vi "Get Comment.vi"(8 "error in (no error)":errorcluster, 11 "Device in":refnum<class "Device.lvclass">) -> (0 "error out":errorcluster, 2 "Comment":string, 3 "Device out":refnum<class "Device.lvclass">)   [LabVIEW 2020, in "HAL.lvlib" / "Device.lvclass"]
uses:
  Device.lvclass
  Device.lvclass/Device.ctl
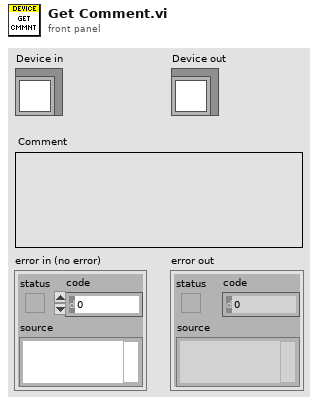
[diagram p1: front panel]
types:
  T1 = typedef "HAL.lvlib/Device.lvclass/Ref Data.ctl" = cluster{"Config Keys":string[], "Config Values":string[], "Cal Expires":timestamp, "Name":string, "Comment":string, "State":T2, "Error":errorcluster}
  T2 = typedef "HAL.lvlib/Device.lvclass/Device State.ctl" = enum16{"Uninitialized", "Initialized", "Ready", "Running", "Error"}
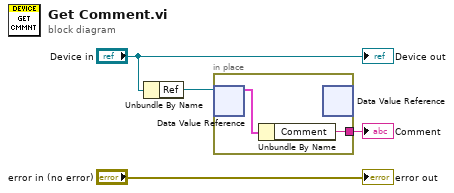
[diagram p0: block diagram]
diagram:
  n1 = Unbundle By Name("Device in") -> ("Ref"=w3:refnum<data-value>)
  n2 = in-place {
    in-place-border: [w6] -> w1
    n3 = in-place-dvr #1(w3) -> (w5:T1)  [unwired: 1 out]
    n4 = Unbundle By Name(w5) -> ("Comment"=w6:string)
    n5 = in-place-dvr #1() -> ()  [unwired: 1 in, 2 out]
  }
  "Comment" <- w1
  "error out" <- "error in (no error)"
  "Device out" <- "Device in"
